vi "Read Owning VI.vi"(8 "error in (no error)":errorcluster, 11 "Generic.lvclass in":refnum<class "Generic.lvclass">) -> (0 "error out":errorcluster, 2 "OwningVI":refnum<vi>, 3 "Generic.lvclass out":refnum<class "Generic.lvclass">)   [LabVIEW 2015, in "Generic.lvclass"]
uses:
  Generic.lvclass
  Generic.lvclass/Generic.ctl
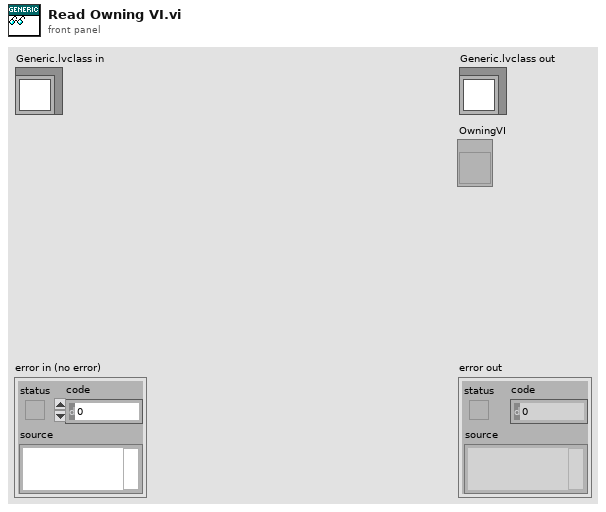
[diagram p1: front panel]
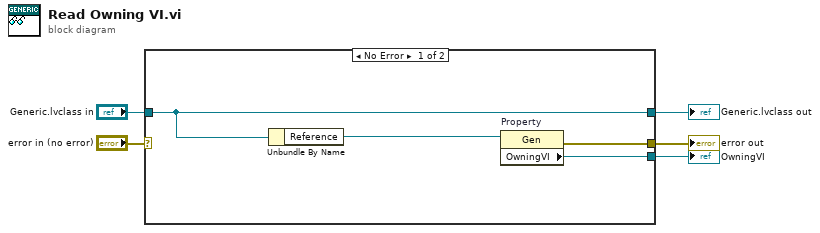
[diagram p0: block diagram]
diagram:
  n1 = case shown="No Error" "error in (no error)" {
    selector: "error in (no error)" -> [_ w11]
    tunnel: [w8 w11] -> w4
    tunnel: [w6 w10] -> w2
    tunnel: "Generic.lvclass in" -> [w6 w10]
    tunnel: [w9 _] -> w1
    frame No Error {
      n2 = Unbundle By Name(w6) -> ("Reference"=w7:refnum<vi>)
      n3 = property on="Property" class="Gen"(reference=w7) -> (error out=w8:errorcluster, "OwningVI"=w9:refnum<vi>)  [unwired: 1 in, 1 out]
    }
    frame Error {
    }
  }
  "error out" <- w4
  "Generic.lvclass out" <- w2
  "OwningVI" <- w1
